vi "VM.vi"(0 "States":refnum<vi>, 1 "algOutputMsgs":refnum<vi>, 3 "INP":refnum<vi>, 4 "PORTS":refnum<vi>, 5 "OUTP":refnum<vi>, 6 "verifier2GUIOutputMsgs":refnum<vi>, 9 "INPUT VARS":refnum<vi>, 10 "Processes":refnum<vi>, 11 "CA2GUI":refnum<vi>, 12 "verifier2scenariousControlOutMsgs":refnum<vi>, 13 "VM2SCM":refnum<vi>, 14 "VM2GUI":refnum<vi>, 15 "VMStates":refnum<vi>) -> ()   [LabVIEW 2019]
uses:
  <vilib>/Utility/miscctls.llb/LVRowAndColumnTypeDef.ctl
panel:
  out "Input messages from CA":T1(array[cluster])
  out "Colors":u32[](array[numeric])
  out "Veriphication results tbl":string[][](table) caption="Verification result"
  in  "Cluster":T2
  out "Array Ports Appended array":i8[](array[numeric])
  out "Output messages to SCM:":T1(array[cluster])
  in  "OUT Ports Array 2":cluster{"Port":string, "Value":bool[]}[](array[cluster]) caption="Input ports values"
  out "Value:":string[](array[string])
  out "Type:":string[](array[string])
  out "Input:":string[](array[string])
  out "States of processes:":string[][](table)
  # "Verification module"
  # "Global variables"
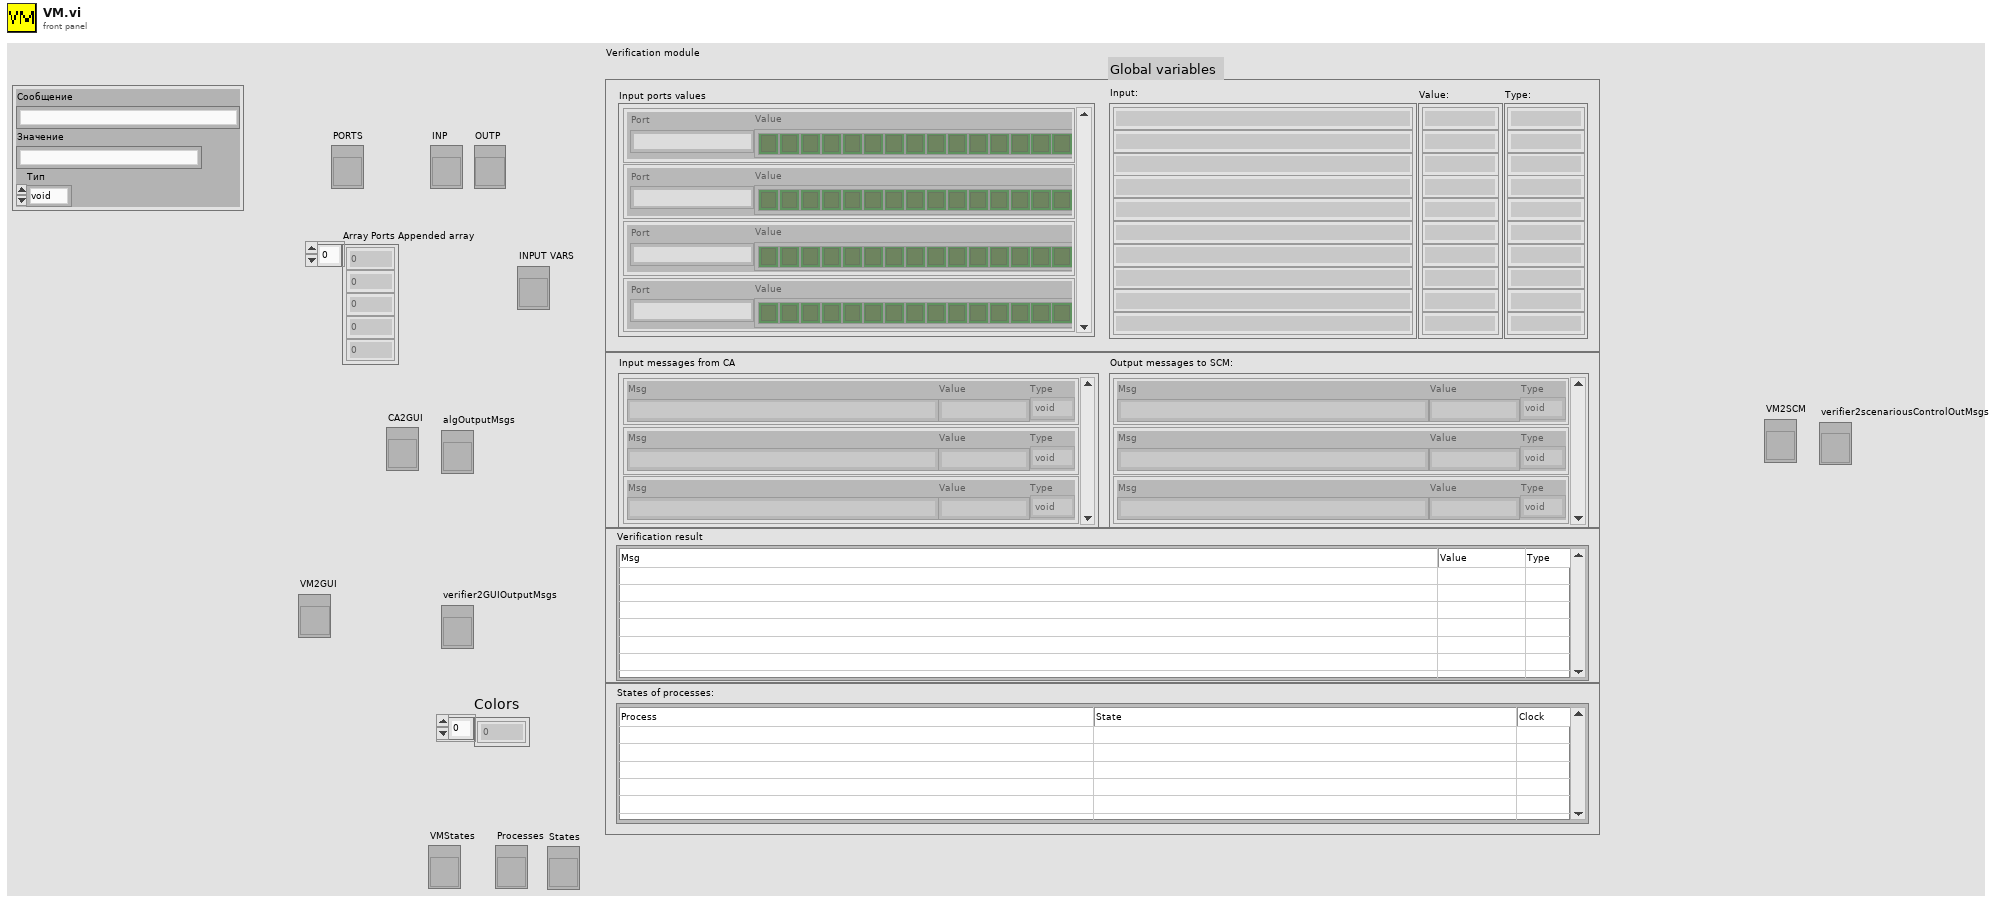
[diagram p1: front panel]
types:
  T1 = cluster{"Msg":string, "Value":string, "Type":enum16{"void", "byte", "int", "float"}}[]
  T2 = cluster{"Сообщение":string, "Значение":string, "Тип":enum16{"void", "byte", "int", "float"}}
  T3 = typedef "LVRowAndColumnTypeDef.ctl" = cluster{"Row":i32, "Column":i32}
  T4 = cluster{"Input varables names":string[], "Input varables type":string[], "Input varables ports":i32[], "Input varables bytes":i32[]}
  T5 = cluster{"Input Numbers":i32[], "Input Names":string[], "Output Names ":string[]}
  T6 = cluster{"Сообщение":string, "Значение":string, "Тип":enum16{"void", "byte", "int", "float"}}[]
  T7 = cluster{"MSG":i16, "param":i32, "Type":enum16{"void", "byte", "int", "float"}}[]
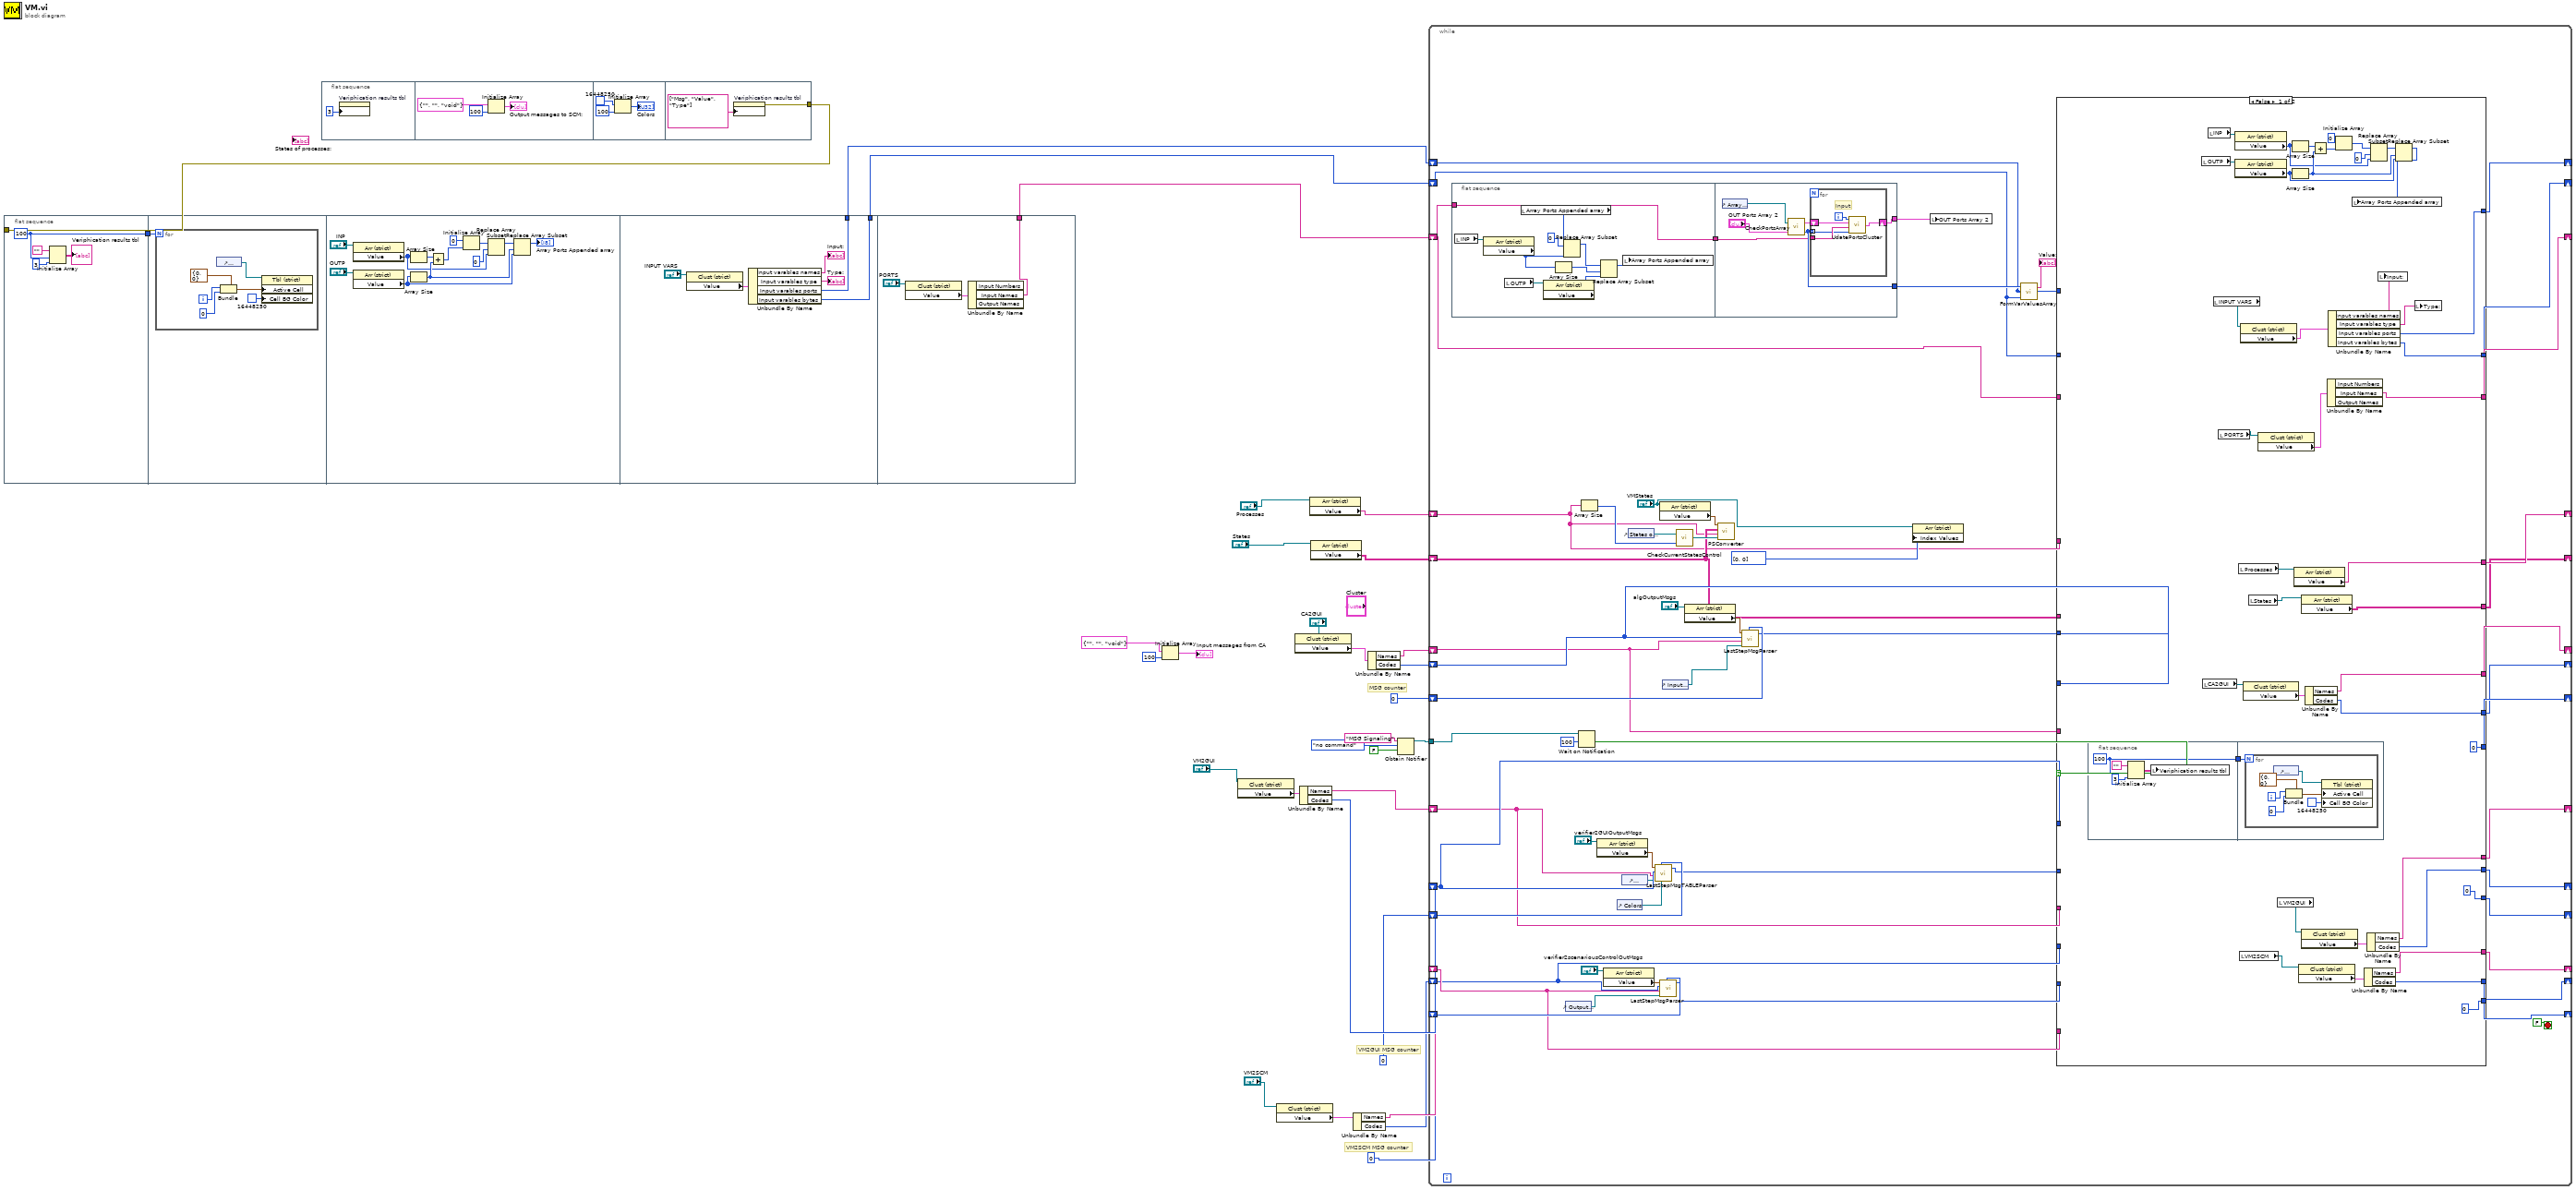
[diagram p0: block diagram]
diagram:
  # "VM2SCM MSG counter"
  # "VM2GUI MSG counter"
  # "MSG counter"
  n1 = flat-sequence {
    tunnel: [w32] -> w5
    tunnel: w4 -> [_]
    tunnel: w5 -> [w36]
    tunnel: [w56] -> w3
    tunnel: [w55] -> w2
    tunnel: [w61] -> w1
    frame #0 {
      w32 = 100 ("dimension size")
      n2 = Initialize Array("", w32, 3 ("dimension size")) -> (→"Veriphication results tbl":string[][])
    }
    frame #1 {
      n3 = for {
        N: w36 -> [_]
        i -> [w41]
        n4 = control-ref of="Veriphication results tbl"() -> (w39:refnum<vi>)
        n5 = Bundle(cluster=T3 {"Row"=0, "Column"=0} ("Active Cell:Active Cell"), "Row"=w41, "Column"=0) -> (w38:T3)
        n6 = property class="Tbl (strict)"(reference=w39, "Active Cell"=w38, "Cell BG Color"=u32 16448250 ("Success")) -> ()  [unwired: 1 in, 2 out]
      }
    }
    frame #2 {
      n7 = property class="Arr (strict)"(reference="INP") -> ("Value"=w45:i8[])  [unwired: 1 in, 2 out]
      n8 = property class="Arr (strict)"(reference="OUTP") -> ("Value"=w44:i8[])  [unwired: 1 in, 2 out]
      n9 = Array Size(array=w45) -> (size(s)=w50:i32)
      n10 = Array Size(array=w44) -> (size(s)=w47:i32)
      n11 = Add(x=w50, y=w47) -> (x+y=w51:i32)
      n12 = Initialize Array(i8 0 ("Numeric"), w51) -> (w49:i8[])
      n13 = Replace Array Subset(array=w49, new element=w45, index=0) -> (w46:i8[])
      n14 = Replace Array Subset(array=w46, new element=w44, index=w47) -> (→"Array Ports Appended array":i8[])
    }
    frame #3 {
      n15 = property class="Clust (strict)"(reference="INPUT VARS") -> ("Value"=w58:T4)  [unwired: 1 in, 2 out]
      n16 = Unbundle By Name(w58) -> ("Input varables names"=→"Input:":string[], "Input varables type"=→"Type:":string[], "Input varables ports"=w56:i32[], "Input varables bytes"=w55:i32[])
    }
    frame #4 {
      n17 = property class="Clust (strict)"(reference="PORTS") -> ("Value"=w63:T5)  [unwired: 1 in, 2 out]
      n18 = Unbundle By Name(w63) -> ("Input Names"=w61:string[])  [unwired: 2 out]
    }
  }
  n19 = flat-sequence {
    tunnel: [w71] -> w4
    frame #0 {
      n20 = property on="Veriphication results tbl" class="Tbl (strict)"("Number of Columns"=u32 3) -> ()  [unwired: 2 in, 2 out]
    }
    frame #1 {
      n21 = Initialize Array(T2 {"Сообщение"="", "Значение"="", "Тип"=enum."void"} ("Cluster"), 100 ("dimension size")) -> (→"Output messages to SCM:":T6)
    }
    frame #2 {
      n22 = Initialize Array(u32 16448250 ("Success"), 100 ("dimension size")) -> (→"Colors":u32[])
    }
    frame #3 {
      n23 = property on="Veriphication results tbl" class="Tbl (strict)"("Column Headers[]"=string[] ["Msg", "Value", "Type"] ("Column Header Strings[]")) -> (error out=w71:errorcluster)  [unwired: 2 in, 1 out]
    }
  }
  n24 = Initialize Array(T2 {"Сообщение"="", "Значение"="", "Тип"=enum."void"} ("Cluster"), 100 ("dimension size")) -> (→"Input messages from CA":T6)
  n25 = property class="Clust (strict)"(reference="VM2GUI") -> ("Value"=w16:cluster{"Names":string[], "Codes":i32[]})  [unwired: 1 in, 2 out]
  n26 = property class="Clust (strict)"(reference="VM2SCM") -> ("Value"=w11:cluster{"Names":string[], "Codes":i32[]})  [unwired: 1 in, 2 out]
  n27 = property class="Clust (strict)"(reference="CA2GUI") -> ("Value"=w26:cluster{"Names":string[], "Codes":i32[]})  [unwired: 1 in, 2 out]
  n28 = Unbundle By Name(w16) -> ("Names"=w14:string[], "Codes"=w13:i32[])
  n29 = property class="Arr (strict)"(reference="Processes") -> ("Value"=w29:string[])  [unwired: 1 in, 2 out]
  n30 = property class="Arr (strict)"(reference="States") -> ("Value"=w28:string[][])  [unwired: 1 in, 2 out]
  n31 = Unbundle By Name(w11) -> ("Names"=w9:string[], "Codes"=w8:i32[])
  n32 = Unbundle By Name(w26) -> ("Names"=w25:string[], "Codes"=w24:i32[])
  n33 = Obtain Notifier(name (unnamed)="MSG Signaling", notification data type=enum16{"no command", "refresh"}."no command", create if not found? (T)=FALSE) -> (notifier out=w17:refnum<notifier>)  [unwired: 1 in, 2 out]
  n34 = while {
    shift-right: [w113] -> _
    shift-left: 0 ("dimension size") -> [w119]
    tunnel: w17 -> [w116]
    shift-right: [w111] -> _
    shift-left: w24 -> [w112]
    shift-right: [w110] -> _
    shift-left: w25 -> [w109]
    shift-right: [w104] -> _
    shift-left: w28 -> [w107]
    shift-right: [w105] -> _
    shift-left: w29 -> [w106]
    shift-right: [w98] -> _
    shift-left: w2 -> [w102]
    shift-right: [w99] -> _
    shift-left: w3 -> [w103]
    shift-right: [w100] -> _
    shift-left: w1 -> [w101]
    shift-right: [w93] -> _
    shift-left: w14 -> [w77]
    shift-right: [w92] -> _
    shift-left: w13 -> [w78]
    shift-right: [w91] -> _
    shift-left: 0 ("dimension size") -> [w80]
    shift-right: [w83] -> _
    shift-left: w9 -> [w85]
    shift-right: [w82] -> _
    shift-left: w8 -> [w84]
    shift-right: [w81] -> _
    shift-left: 0 ("dimension size") -> [w87]
    stop <- FALSE ("stop") stop-if-true
    n35 = flat-sequence {
      tunnel: w101 -> [w137]
      tunnel: [w137] -> w95
      tunnel: [w142] -> w118
      tunnel: [w139] -> w96
      tunnel: w95 -> [w141]
      frame #0 {
        n36 = local read "INP"() -> (w128:refnum<vi>)
        n37 = property class="Arr (strict)"(reference=w128) -> ("Value"=w136:i8[])  [unwired: 1 in, 2 out]
        n38 = local read "OUTP"() -> (w129:refnum<vi>)
        n39 = local read "Array Ports Appended array"() -> (w133:i8[])
        n40 = property class="Arr (strict)"(reference=w129) -> ("Value"=w135:i8[])  [unwired: 1 in, 2 out]
        n41 = Array Size(array=w136) -> (size(s)=w132:i32)
        n42 = Replace Array Subset(array=w133, new element=w136, index=0) -> (w131:i8[])
        n43 = Replace Array Subset(array=w131, new element=w135, index=w132) -> (w134:i8[])
        n44 = local write "Array Ports Appended array"(w134) -> ()
      }
      frame #1 {
        n45 = control-ref of="Array Ports Appended array"() -> (w138:refnum<vi>)
        n46 = call "CheckPortsArray.vi"("INP Ports Array 2"="OUT Ports Array 2", "INP"=w138) -> ("Value"=w142:i8[], "INP Ports Array"=w143:cluster{"String":string, "Array 2":bool[]}[])
        n47 = for {
          tunnel: w142 -> [w147] mode=indexing
          tunnel: w141 -> [w148]
          shift-right: [w144] -> w139
          shift-left: w143 -> [w145]
          i -> [w146]
          # "Input"
          n48 = call "UdatePortsCluster.vi"("Numeric 2"=w147, "Input Names"=w148, "Ports Array"=w145, "index"=w146) -> ("INP Ports Array 2"=w144:cluster{"String":string, "Array 2":bool[]}[])
        }
      }
    }
    n49 = control-ref of="Output messages to SCM:"() -> (w88:refnum<vi>)
    n50 = Wait on Notification(notifier=w116, timeout in ms (-1)=100) -> (timed out?=w115:bool)  [unwired: 2 in, 3 out]
    n51 = Array Size(array=w106) -> (size(s)=w108:i32)
    n52 = property class="Arr (strict)"(reference="verifier2GUIOutputMsgs") -> ("Value"=w79:cluster{"MSG":i16, "param":i32, "Type":i16}[])  [unwired: 1 in, 2 out]
    n53 = property class="Arr (strict)"(reference="verifier2scenariousControlOutMsgs") -> ("Value"=w90:cluster{"MSG":i16, "param":i32, "Type":i16}[])  [unwired: 1 in, 2 out]
    n54 = control-ref of="Colors"() -> (w74:refnum<vi>)
    n55 = control-ref of="Veriphication results tbl"() -> (w76:refnum<vi>)
    n56 = control-ref of="States of processes:"() -> (w126:refnum<vi>)
    n57 = call "LastStepMsgTABLEParser.vi"("Color Arr Refnum"=w74, "Tbl Refnum"=w76, "Out MSG Names"=w77, "old msg counter"=w80, "Codes"=w78, "Msg Array"=w79) -> ("current msg counter"=w75:i32)  [unwired: 3 in, 1 out]
    n58 = property class="Arr (strict)"(reference="VMStates") -> ("Value"=w127:cluster{"TimeInState":u16, "cur_state":i8}[])  [unwired: 1 in, 2 out]
    n59 = call "LastStepMsgParser.vi"("Arr Refnum"=w88, "Out MSG Names"=w85, "old msg counter"=w87, "Codes"=w84, "Msg Array"=w90) -> ("current msg counter"=w86:i32)  [unwired: 4 in, 1 out]
    n60 = control-ref of="Input messages from CA"() -> (w73:refnum<vi>)
    n61 = call "CheckCurrentStatesControl.vi"("Processes"=w108, "Inp reference"=w126) -> ("Out Refnum"=w125:refnum<vi>)
    n62 = property class="Arr (strict)"(reference="algOutputMsgs") -> ("Value"=w120:T7)  [unwired: 1 in, 2 out]
    n63 = call "PSConverter.vi"("Tbl Refnum"=w125, "PROC"=w106, "STATES"=w107, "Input claster"=w127) -> ()  [unwired: 1 out]
    n64 = call "LastStepMsgParser.vi"("Arr Refnum"=w73, "Out MSG Names"=w109, "old msg counter"=w119, "Codes"=w112, "Msg Array"=w120) -> ("current msg counter"=w114:i32)  [unwired: 4 in, 1 out]
    n65 = property class="Arr (strict)"(reference="VMStates", "Index Values"=u32[] [0, 0]) -> ()  [unwired: 1 in, 2 out]
    n66 = local write "OUT Ports Array 2"(w96) -> ()
    n67 = call "FormVarValuesArray.vi"("varables bytes"=w102, "varables ports"=w103, "Ports"=w118) -> ("Values Array"=→"Value:":string[])  [unwired: 1 in]
    n68 = case shown="False" w115 {
      tunnel: w114 -> [_ w212]
      tunnel: [0 ("current msg counter") w212] -> w113
      tunnel: w112 -> [_ w214]
      tunnel: [w185 w214] -> w111
      tunnel: [w186 w213] -> w110
      tunnel: w109 -> [_ w213]
      tunnel: w107 -> [_ w210]
      tunnel: w106 -> [_ w211]
      tunnel: [w183 w211] -> w105
      tunnel: [w181 w210] -> w104
      tunnel: w103 -> [_ w208]
      tunnel: w102 -> [_ w207]
      tunnel: w101 -> [_ w209]
      tunnel: [w162 w209] -> w100
      tunnel: [w176 w208] -> w99
      tunnel: [w177 w207] -> w98
      tunnel: w77 -> [_ w205]
      tunnel: w75 -> [_ w206]
      tunnel: [w159 w205] -> w93
      tunnel: [w158 w201] -> w92
      tunnel: [0 ("current msg counter") w206] -> w91
      tunnel: w86 -> [_ w203]
      tunnel: w85 -> [_ w202]
      tunnel: w84 -> [_ w204]
      tunnel: [w154 w202] -> w83
      tunnel: [w153 w204] -> w82
      tunnel: [0 ("current msg counter") w203] -> w81
      tunnel: w78 -> [_ w201]
      frame False {
        n69 = flat-sequence {
          tunnel: [w190] -> w151
          tunnel: w151 -> [w194]
          frame #0 {
            w190 = 100 ("dimension size")
            n70 = Initialize Array("", w190, 3 ("dimension size")) -> (w193:string[][])
            n71 = local write "Veriphication results tbl"(w193) -> ()
          }
          frame #1 {
            n72 = for {
              N: w194 -> [_]
              i -> [w199]
              n73 = control-ref of="Veriphication results tbl"() -> (w195:refnum<vi>)
              n74 = Bundle(cluster=T3 {"Row"=0, "Column"=0} ("Active Cell:Active Cell"), "Row"=w199, "Column"=0) -> (w197:T3)
              n75 = property class="Tbl (strict)"(reference=w195, "Active Cell"=w197, "Cell BG Color"=u32 16448250 ("Success")) -> ()  [unwired: 1 in, 2 out]
            }
          }
        }
        n76 = local read "OUTP"() -> (w165:refnum<vi>)
        n77 = local read "CA2GUI"() -> (w188:refnum<vi>)
        n78 = local read "INP"() -> (w166:refnum<vi>)
        n79 = local read "INPUT VARS"() -> (w178:refnum<vi>)
        n80 = local read "PORTS"() -> (w180:refnum<vi>)
        n81 = property class="Arr (strict)"(reference=w166) -> ("Value"=w168:i8[])  [unwired: 1 in, 2 out]
        n82 = property class="Arr (strict)"(reference=w165) -> ("Value"=w167:i8[])  [unwired: 1 in, 2 out]
        n83 = local read "Processes"() -> (w184:refnum<vi>)
        n84 = local read "VM2SCM"() -> (w155:refnum<vi>)
        n85 = property class="Clust (strict)"(reference=w178) -> ("Value"=w179:T4)  [unwired: 1 in, 2 out]
        n86 = property class="Clust (strict)"(reference=w188) -> ("Value"=w187:cluster{"Names":string[], "Codes":i32[]})  [unwired: 1 in, 2 out]
        n87 = local read "States"() -> (w182:refnum<vi>)
        n88 = property class="Clust (strict)"(reference=w180) -> ("Value"=w163:T5)  [unwired: 1 in, 2 out]
        n89 = local read "VM2GUI"() -> (w161:refnum<vi>)
        n90 = Array Size(array=w168) -> (size(s)=w173:i32)
        n91 = Array Size(array=w167) -> (size(s)=w170:i32)
        n92 = property class="Arr (strict)"(reference=w184) -> ("Value"=w183:string[])  [unwired: 1 in, 2 out]
        n93 = property class="Clust (strict)"(reference=w155) -> ("Value"=w156:cluster{"Names":string[], "Codes":i32[]})  [unwired: 1 in, 2 out]
        n94 = property class="Arr (strict)"(reference=w182) -> ("Value"=w181:string[][])  [unwired: 1 in, 2 out]
        n95 = property class="Clust (strict)"(reference=w161) -> ("Value"=w160:cluster{"Names":string[], "Codes":i32[]})  [unwired: 1 in, 2 out]
        n96 = Unbundle By Name(w187) -> ("Names"=w186:string[], "Codes"=w185:i32[])
        n97 = Add(x=w173, y=w170) -> (x+y=w174:i32)
        n98 = Unbundle By Name(w163) -> ("Input Names"=w162:string[])  [unwired: 2 out]
        n99 = Unbundle By Name(w179) -> ("Input varables names"=w150:string[], "Input varables type"=w149:string[], "Input varables ports"=w176:i32[], "Input varables bytes"=w177:i32[])
        n100 = Initialize Array(i8 0 ("Numeric"), w174) -> (w172:i8[])
        n101 = Unbundle By Name(w156) -> ("Names"=w154:string[], "Codes"=w153:i32[])
        n102 = Unbundle By Name(w160) -> ("Names"=w159:string[], "Codes"=w158:i32[])
        n103 = Replace Array Subset(array=w172, new element=w168, index=0) -> (w169:i8[])
        n104 = local write "Input:"(w150) -> ()
        n105 = Replace Array Subset(array=w169, new element=w167, index=w170) -> (w164:i8[])
        n106 = local write "Array Ports Appended array"(w164) -> ()
        n107 = local write "Type:"(w149) -> ()
      }
      frame True {
      }
    }
  }
